vi "LOGIC_LibGetStats.vi"(7 "bpp":i32, 10 "num_elems":u32, 11 "imageptr":u64) -> (1 "var":sgl, 2 "mean":sgl)   [LabVIEW 2016]
uses:
  public/c/lib/libLogic.so
panel:
  in  "stats":sgl[](array[numeric])=[0.0, 0.0, 0.0, 0.0, 0.0]
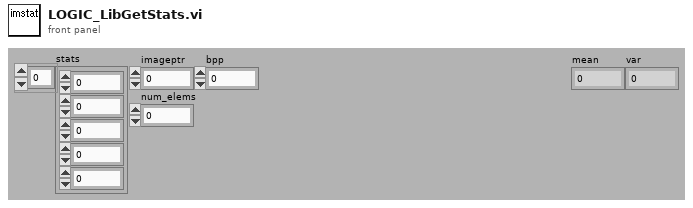
[diagram p1: front panel]
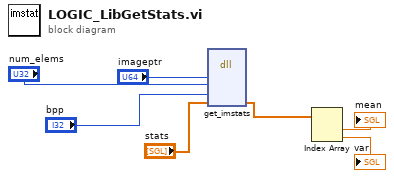
[diagram p0: block diagram]
diagram:
  n1 = dll-call lib="home/simager/panview/PAN/Modules/Logical/public/c/lib/libLogic.so" fn="get_imstats"("imageptr"="imageptr", "num_elems"="num_elems", "bpp"="bpp", "stats"="stats") -> ("stats"=w3:sgl[])  [unwired: 6 in, 3 out]
  n2 = Index Array(array=w3) -> (element #1=→"mean":sgl, element #2=→"var":sgl)  [unwired: 2 in]
